vi "Single-Thumbstick Drive.vi"(2 "X-Input":dbl(slide) scale=-1.0..1.0, 3 "Y-Input":dbl(slide) scale=-1.0..1.0) -> (0 "Right":dbl(slide) scale=-1.0..1.0, 1 "Left":dbl(slide) scale=-1.0..1.0)   [LabVIEW 2011]
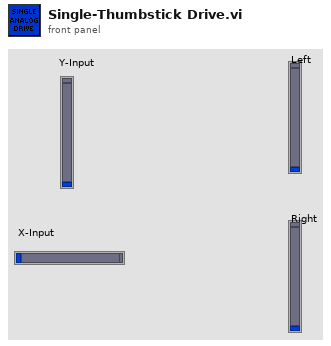
[diagram p1: front panel]
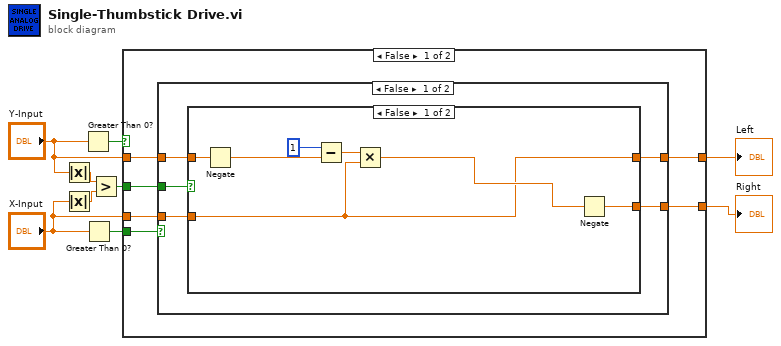
[diagram p0: block diagram]
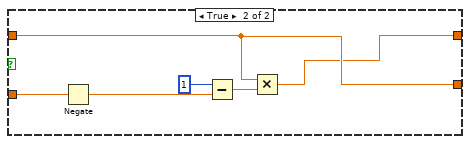
[diagram p2: hidden frame]
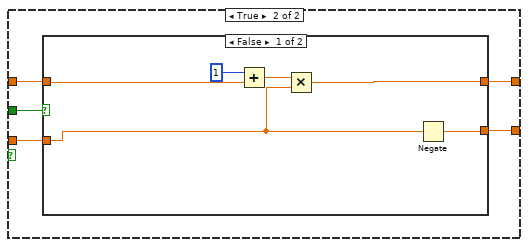
[diagram p3: hidden frame]
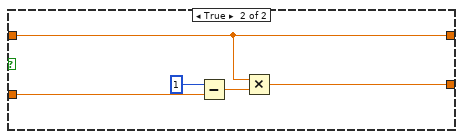
[diagram p4: hidden frame]
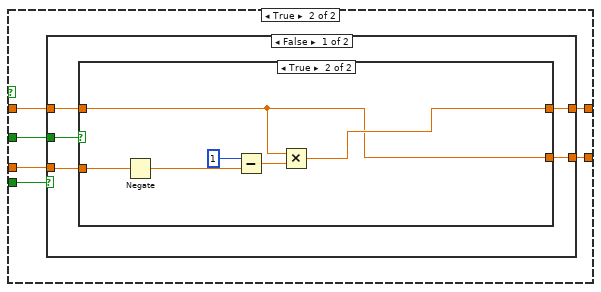
[diagram p5: hidden frame]
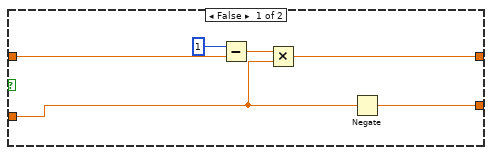
[diagram p6: hidden frame]
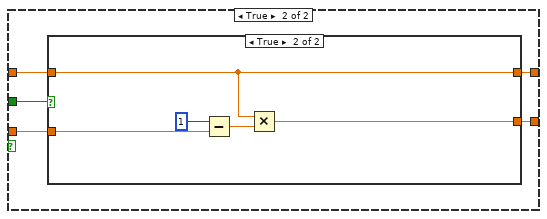
[diagram p7: hidden frame]
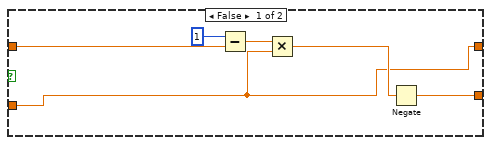
[diagram p8: hidden frame]
diagram:
  n1 = Absolute Value(x="Y-Input") -> (abs(x)=w7:dbl)
  n2 = Absolute Value(x="X-Input") -> (abs(x)=w6:dbl)
  n3 = Greater Than 0?(x="Y-Input") -> (x > 0?=w9:bool)
  n4 = Greater Than 0?(x="X-Input") -> (x > 0?=w8:bool)
  n5 = Greater?(x=w7, y=w6) -> (0:w5:bool)
  n6 = case shown="False" w9 {
    tunnel: w8 -> [w15 w55]
    tunnel: w5 -> [w14 w54]
    tunnel: [w12 w53] -> w4
    tunnel: "Y-Input" -> [w11 w52]
    tunnel: "X-Input" -> [w10 w51]
    tunnel: [w13 w50] -> w1
    frame False {
      n7 = case shown="False" w15 {
        tunnel: w14 -> [w20 w38]
        tunnel: [w19 w37] -> w13
        tunnel: [w18 w36] -> w12
        tunnel: w11 -> [w17 w35]
        tunnel: w10 -> [w16 w34]
        frame False {
          n8 = case shown="False" w20 {
            tunnel: [w21 w30] -> w19
            tunnel: [w22 w28] -> w18
            tunnel: w17 -> [w27 w30]
            tunnel: w16 -> [w22 w31]
            frame False {
              n9 = Negate(x=w27) -> (-x=w25:dbl)
              n10 = Subtract(x=1, y=w25) -> (x-y=w24:dbl)
              n11 = Multiply(x=w24, y=w22) -> (x*y=w23:dbl)
              n12 = Negate(x=w23) -> (-x=w21:dbl)
            }
            frame True {
              n13 = Negate(x=w31) -> (-x=w29:dbl)
              n14 = Subtract(x=1, y=w29) -> (x-y=w32:dbl)
              n15 = Multiply(x=w30, y=w32) -> (x*y=w28:dbl)
            }
          }
        }
        frame True {
          n16 = case shown="False" w38 {
            tunnel: [w39 w47] -> w37
            tunnel: [w40 w45] -> w36
            tunnel: w35 -> [w42 w45]
            tunnel: w34 -> [w41 w46]
            frame False {
              n17 = Add(x=1, y=w42) -> (x+y=w44:dbl)
              n18 = Multiply(x=w44, y=w41) -> (x*y=w40:dbl)
              n19 = Negate(x=w41) -> (-x=w39:dbl)
            }
            frame True {
              n20 = Subtract(x=1, y=w46) -> (x-y=w48:dbl)
              n21 = Multiply(x=w45, y=w48) -> (x*y=w47:dbl)
            }
          }
        }
      }
    }
    frame True {
      n22 = case shown="False" w55 {
        tunnel: w54 -> [w60 w77]
        tunnel: [w59 w76] -> w53
        tunnel: w52 -> [w58 w75]
        tunnel: w51 -> [w57 w74]
        tunnel: [w56 w73] -> w50
        frame False {
          n23 = case shown="True" w60 {
            tunnel: [w61 w70] -> w59
            tunnel: w58 -> [w63 w69]
            tunnel: w57 -> [w64 w67]
            tunnel: [w62 w69] -> w56
            frame False {
              n24 = Subtract(x=1, y=w63) -> (x-y=w66:dbl)
              n25 = Multiply(x=w66, y=w64) -> (x*y=w61:dbl)
              n26 = Negate(x=w64) -> (-x=w62:dbl)
            }
            frame True {
              n27 = Negate(x=w67) -> (-x=w68:dbl)
              n28 = Subtract(x=1, y=w68) -> (x-y=w72:dbl)
              n29 = Multiply(x=w69, y=w72) -> (x*y=w70:dbl)
            }
          }
        }
        frame True {
          n30 = case shown="True" w77 {
            tunnel: [w79 w85] -> w76
            tunnel: w75 -> [w82 w85]
            tunnel: w74 -> [w79 w87]
            tunnel: [w78 w84] -> w73
            frame False {
              n31 = Subtract(x=1, y=w82) -> (x-y=w81:dbl)
              n32 = Multiply(x=w81, y=w79) -> (x*y=w80:dbl)
              n33 = Negate(x=w80) -> (-x=w78:dbl)
            }
            frame True {
              n34 = Subtract(x=1, y=w87) -> (x-y=w86:dbl)
              n35 = Multiply(x=w85, y=w86) -> (x*y=w84:dbl)
            }
          }
        }
      }
    }
  }
  "Left" <- w4
  "Right" <- w1
